vi "S2C_Shared_Proc_OpenRefs.vi"(8 "Error In":errorcluster, 11 "VI_Ref":refnum<vi>) -> (0 "Error Out":errorcluster, 3 "Refs":string[][](array[string]))   [LabVIEW 2015]
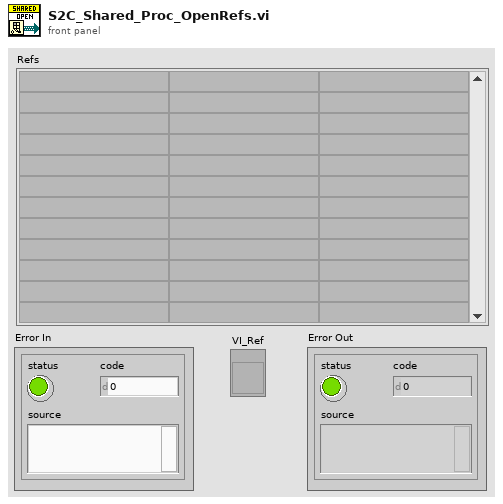
[diagram p1: front panel]
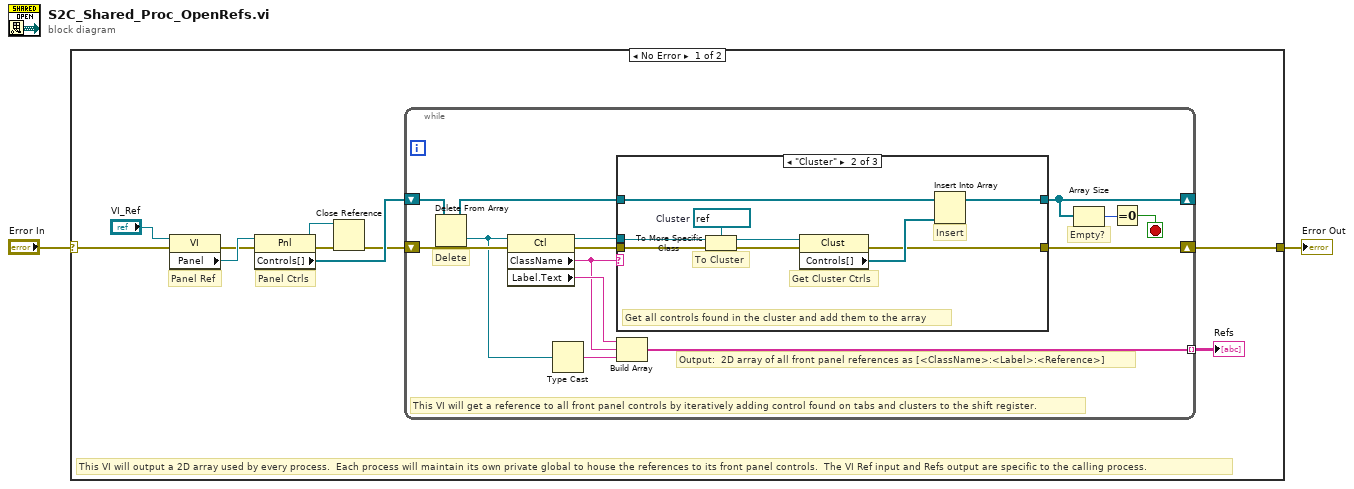
[diagram p0: block diagram]
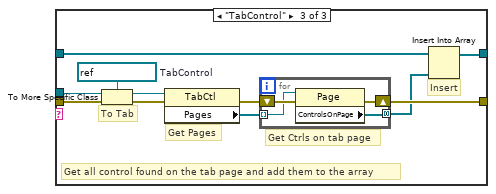
[diagram p3: hidden frame]
diagram:
  n1 = case shown="No Error" "Error In" {
    selector: "Error In" -> [w8 w53]
    tunnel: [w7 w53] -> w1
    frame No Error {
      # "This VI will output a 2D array used by every process.  Each process will maintain its own private global to house the references to its front panel controls.  The VI Ref input and Refs output are specific to the calling process."
      # "Panel Ctrls"
      # "Panel Ref"
      n2 = property class="VI"(reference="VI_Ref", error in=w8) -> (error out=w11:errorcluster, "Panel"=w12:refnum<vi>)  [unwired: 1 out]
      n3 = property class="Pnl"(reference=w12, error in=w11) -> (reference out=w3:refnum<vi>, error out=w5:errorcluster, "Controls[]"=w10:refnum<vi>[])
      n4 = Close Reference(reference=w3, error in (no error)=w5) -> (error out=w4:errorcluster)
      n5 = while {
        shift-right: [w21] -> _
        shift-left: w10 -> [w25]
        shift-right: [w23] -> w7
        shift-left: w4 -> [w26]
        tunnel: [w18] -> w6 mode=indexing
        stop <- w19 stop-if-true
        # "Empty?"
        # "Output:  2D array of all front panel references as [<ClassName>:<Label>:<Reference>]"
        # "This VI will get a reference to all front panel controls by iteratively adding control found on tabs and clusters to the shift register."
        # "Delete"
        n6 = Delete From Array(array=w25) -> (deleted portion=w13:refnum<vi>, array with subset deleted=w22:refnum<vi>[])  [unwired: 2 in]
        n7 = property class="Ctl"(reference=w13, error in=w26) -> (reference out=w14:refnum<vi>, error out=w24:errorcluster, "ClassName"=w16:string, "Label.Text"=w17:string)
        n8 = Type Cast(x=w13) -> (*(type *) &x=w15:string)  [unwired: 1 in]
        n9 = case shown="\"Cluster\"" w16 {
          tunnel: w14 -> [_ w36 w47]
          tunnel: w22 -> [w28 w32 w43]
          tunnel: [w28 w30 w42] -> w21
          tunnel: w24 -> [w27 w37 w48]
          tunnel: [w27 w29 w39] -> w23
          frame "Other", Default {
            # "Not Cluster or Tab control"
          }
          frame "Cluster" {
            w35 = refnum<vi> refnum  # Cluster
            # "Get all controls found in the cluster and add them to the array"
            # "Get Cluster Ctrls"
            # "To Cluster"
            # "Insert"
            n10 = To More Specific Class(target class=w35, reference=w36, error in=w37) -> (specific class reference=w33:refnum<vi>, error out=w34:errorcluster)
            n11 = property class="Clust"(reference=w33, error in=w34) -> (error out=w29:errorcluster, "Controls[]"=w31:refnum<vi>[])  [unwired: 1 out]
            n12 = Insert Into Array(array=w32, new element=w31) -> (w30:refnum<vi>[])  [unwired: 1 in]
          }
          frame "TabControl" {
            w46 = refnum<vi> refnum  # TabControl
            # "Get all control found on the tab page and add them to the array"
            # "Insert"
            # "Get Ctrls on tab page"
            # "Get Pages"
            # "To Tab"
            n13 = To More Specific Class(target class=w46, reference=w47, error in=w48) -> (specific class reference=w44:refnum<vi>, error out=w45:errorcluster)
            n14 = property class="TabCtl"(reference=w44, error in=w45) -> (error out=w40:errorcluster, "Pages"=w41:refnum<vi>[])  [unwired: 1 out]
            n15 = for {
              tunnel: w41 -> [w51] mode=indexing
              shift-right: [w49] -> w39
              shift-left: w40 -> [w52]
              tunnel: [w50] -> w38 mode=concatenating
              n16 = property class="Page"(reference=w51, error in=w52) -> (error out=w49:errorcluster, "ControlsOnPage"=w50:refnum<vi>[])  [unwired: 1 out]
            }
            n17 = Insert Into Array(array=w43, new element=w38) -> (w42:refnum<vi>[])  [unwired: 1 in]
          }
        }
        n18 = Build Array(w17, w16, w15) -> (w18:string[])
        n19 = Array Size(array=w21) -> (size(s)=w20:i32)
        n20 = Equal To 0?(x=w20) -> (x = 0?=w19:bool)
      }
      "Refs" <- w6
    }
    frame Error {
    }
  }
  "Error Out" <- w1
